vi "Driver - DTACQ - Read Single Line.vi"(8 "error in":errorcluster, 11 "DTACQ Connection Data In":T1={"Description"="", "Address"="", "Port"=0, "timeout (ms)"=5000, "Termination Character"="\n", "TCP Connection Reference"=refnum, "Open Connection"=FALSE}) -> (0 "error out":errorcluster, 1 "Timed Out":bool, 2 "Read String":string, 3 "DTACQ Connection Data Out":T1={"Description"="", "Address"="", "Port"=0, "timeout (ms)"=5000, "Termination Character"="\n", "TCP Connection Reference"=refnum, "Open Connection"=FALSE})   [LabVIEW 2017, in "Communications Library.lvlib"]
doc: "Clears any characters in the read buffer."
uses:
  Communications Library.lvlib
  Typedefs/DTACQ Connection Data--Cluster.ctl
  Debug - Lower Level - Logging Tool.vi
  Error 5102 - DTACQ unit replied with an error--const.vi
  <vilib>/Utility/error.llb/Error Cluster From Error Code.vi
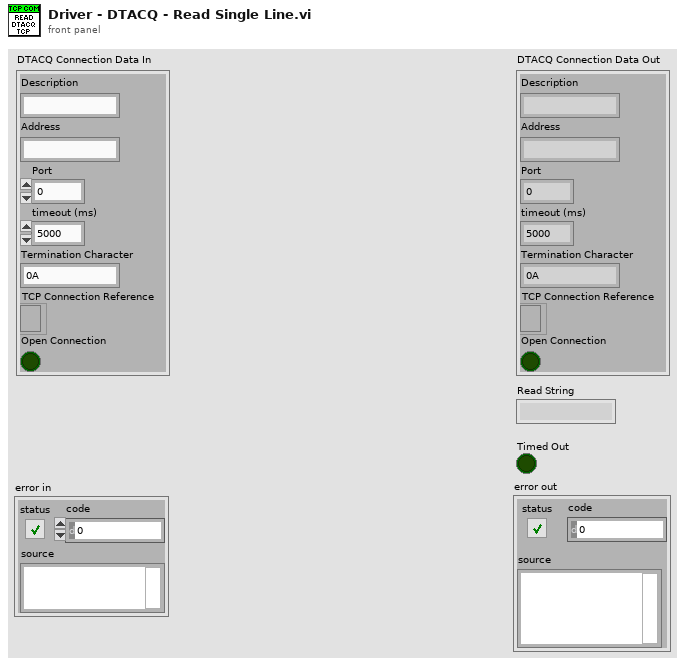
[diagram p1: front panel]
types:
  T1 = typedef "Communications Library.lvlib/DTACQ Connection Data--Cluster.ctl" = cluster{"Description":string, "Address":string, "Port":u16, "timeout (ms)":i32, "Termination Character":string, "TCP Connection Reference":refnum<k5>, "Open Connection":bool}
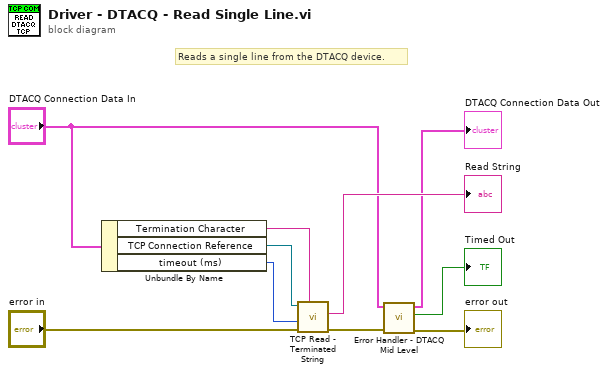
[diagram p0: block diagram]
diagram:
  # "Reads a single line from the DTACQ device."
  n1 = Unbundle By Name("DTACQ Connection Data In") -> ("Termination Character"=w7:string, "TCP Connection Reference"=w9:refnum<k5>, "timeout (ms)"=w8:i32)
  n2 = call "TCP Read - Terminated String.vi"("Termination Character"=w7, "error in"="error in", "Timeout ms (default 50ms)"=w8, "TCP Network Connection in"=w9) -> ("error out"=w5:errorcluster, "Read String"=→"Read String":string)  [unwired: 5 in, 1 out]
  n3 = call "Error Handler - DTACQ Mid Level.vi"("error in"=w5, "DTACQ Connection Data In"="DTACQ Connection Data In") -> ("error out"=→"error out":errorcluster, "Timed Out"=→"Timed Out":bool, "DTACQ Connection Data Out"=→"DTACQ Connection Data Out":T1)  [unwired: 7 in]
